vi "Main.vi"() -> ()   [LabVIEW 2011]
uses:
  Ch1.ctl
  <vilib>/DAQmx/write.llb/DAQmx Write (Analog DBL 1Chan 1Samp).vi
  <vilib>/DAQmx/read.llb/DAQmx Read (Analog DBL 1Chan 1Samp).vi
  <vilib>/DAQmx/write.llb/DAQmx Write (Digital Bool 1Line 1Point).vi
  <vilib>/DAQmx/read.llb/DAQmx Read (Digital Bool 1Line 1Point).vi
  <vilib>/DAQmx/create/channels.llb/DAQmx Create Channel (AO-Voltage-Basic).vi
  <vilib>/DAQmx/create/channels.llb/DAQmx Create Channel (AI-Voltage-Basic).vi
  <vilib>/DAQmx/create/channels.llb/DAQmx Create Channel (DO-Digital Output).vi
  <vilib>/DAQmx/create/channels.llb/DAQmx Create Channel (DI-Digital Input).vi
  <vilib>/DAQmx/miscellaneous.llb/DAQmx Fill In Error Info.vi
panel:
  out "P1.3":bool
  out "P1.2":bool
  out "P1.1":bool
  out "P1.0":bool
  in  "P0.3":bool
  in  "P0.2":bool
  in  "P0.1":bool
  in  "P0.0":bool
  out "U04, B":refnum<k21>
  out "U37, B":refnum<k21>
  out "U26, B":refnum<k21>
  out "U15, B":refnum<k21>
  in  "U1, B":dbl format="%0.2f"
  in  "U0, B":dbl format="%0.2f"
  in  "Зчитати з  P1.3":bool
  in  "Зчитати з  P1.2":bool
  in  "Зчитати з  P1.1":bool
  in  "Зчитати з  P1.0":bool
  in  "Записати в P0.3":bool
  in  "Записати в P0.2":bool
  in  "Записати в P0.1":bool
  in  "Записати в P0.0":bool
  in  "Зчитати з  Аl 37 (3)":bool
  in  "Зчитати з  Аl 26 (2)":bool
  in  "Зчитати з  Аl 15 (1)":bool
  in  "Зчитати з  Аl 04 (0)":bool
  in  "Записати в АО 1":bool
  in  "Записати в АО 0":bool
  in  "Exit":bool
  # "Аналогові канали"
  # "Цифрові канали"
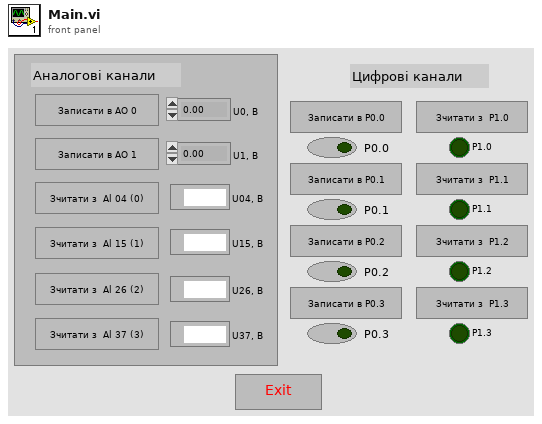
[diagram p1: front panel]
types:
  T1 = typedef "Ch1.ctl" = enum16{"def", "Exit", "Записати в АО 0", "Записати в АО 1", "Зчитати з  Аl 04 (0)", "Зчитати з  Аl 15 (1)", "Зчитати з  Аl 26 (2)", "Зчитати з  Аl 37 (3)", "Записати в P0.0", "Записати в  P0.1", "Записати в P0.2", "Записати в P0.3", "Зчитати з  P1.0", "Зчитати з  P1.1", "Зчитати з  P1.2", "Зчитати з  P1.3"}
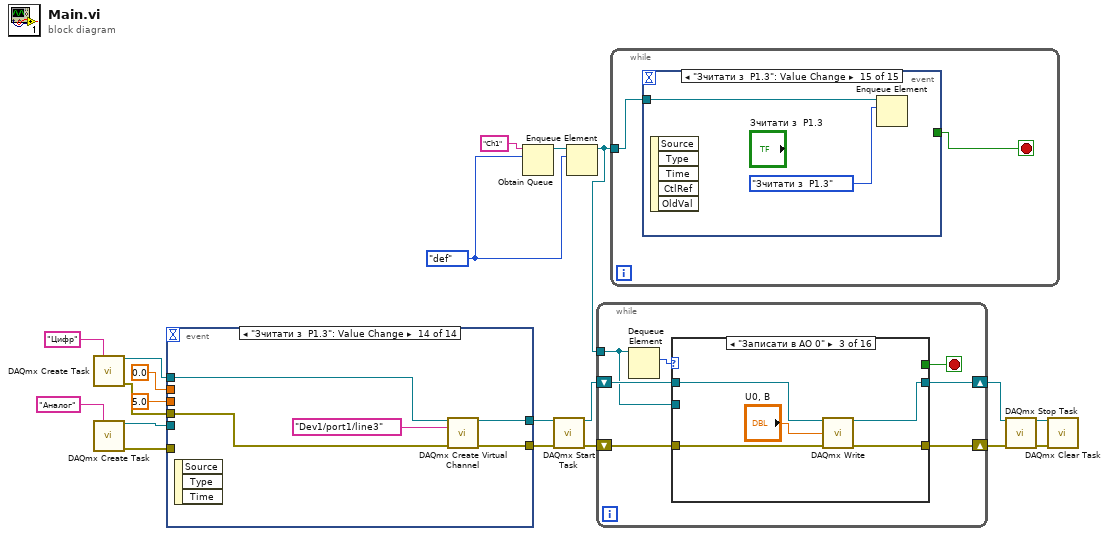
[diagram p0: block diagram]
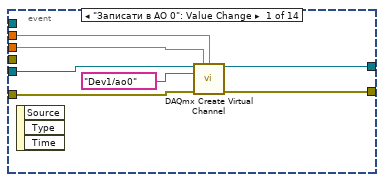
[diagram p2: hidden frame]
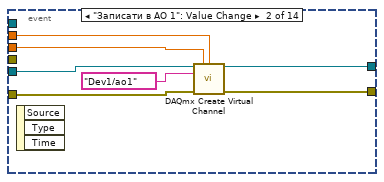
[diagram p3: hidden frame]
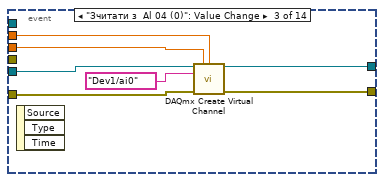
[diagram p4: hidden frame]
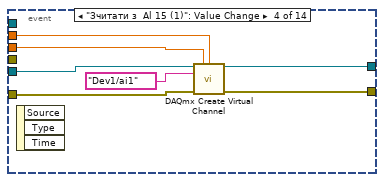
[diagram p5: hidden frame]
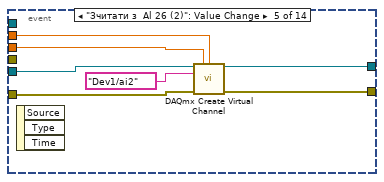
[diagram p6: hidden frame]
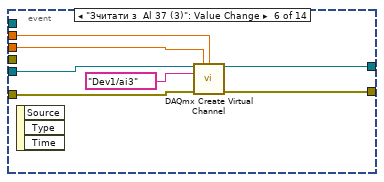
[diagram p7: hidden frame]
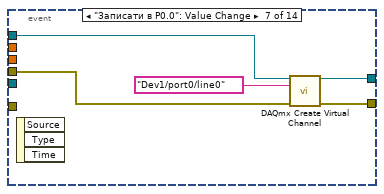
[diagram p8: hidden frame]
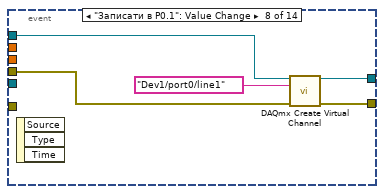
[diagram p9: hidden frame]
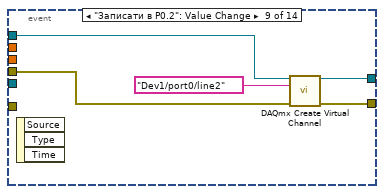
[diagram p10: hidden frame]
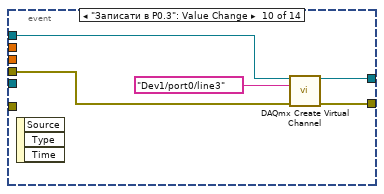
[diagram p11: hidden frame]
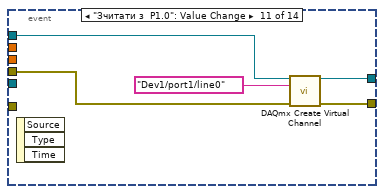
[diagram p12: hidden frame]
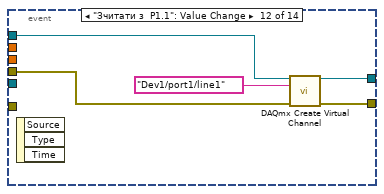
[diagram p13: hidden frame]
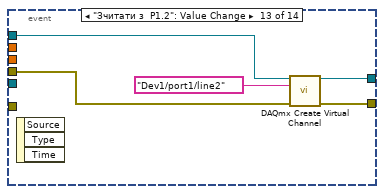
[diagram p14: hidden frame]
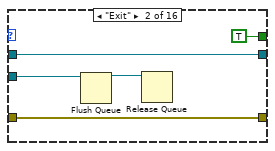
[diagram p16: hidden frame]
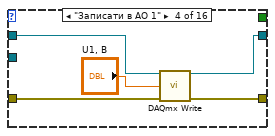
[diagram p17: hidden frame]
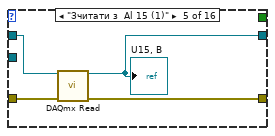
[diagram p18: hidden frame]
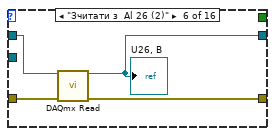
[diagram p19: hidden frame]
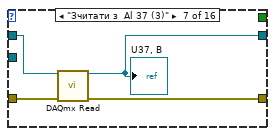
[diagram p20: hidden frame]
diagram:
  w20 = Ch1."def" ("Enum")
  n1 = call <vilib>:"DAQmx Create Task.vi"("new task name"="Цифр") -> ("task out"=w2:refnum<k21>, "error out"=w1:errorcluster)  [unwired: 13 in]
  n2 = call <vilib>:"DAQmx Create Task.vi"("new task name"="Аналог") -> ("task out"=w9:refnum<k21>, "error out"=w8:errorcluster)  [unwired: 13 in]
  n3 = event shown="[13] \"Зчитати з  P1.3\": Value Change" {
    selector: _ -> [_ _ _ _ _ _ _ _ _ _ _ _ _ _]
    dyn-events: _ -> [_ _ _ _ _ _ _ _ _ _ _ _ _ _]
    timeout: _ -> [_ _ _ _ _ _ _ _ _ _ _ _ _ _]
    tunnel: w9 -> [w26 w33 w41 w48 w55 w62 _ _ _ _ _ _ _ _]
    tunnel: w8 -> [w25 w32 w40 w47 w54 w61 _ _ _ _ _ _ _ _]
    tunnel: [w24 w31 w39 w46 w53 w60 w64 w69 w74 w79 w84 w89 w94 w99] -> w7
    tunnel: [w23 w30 w38 w45 w52 w59 w63 w68 w73 w78 w83 w88 w93 w98] -> w6
    tunnel: 0.0 ("minimum value") -> [w22 w29 w37 w44 w51 w58 _ _ _ _ _ _ _ _]
    tunnel: 5.0 ("maximum value") -> [w21 w28 w36 w43 w50 w57 _ _ _ _ _ _ _ _]
    tunnel: w2 -> [_ _ _ _ _ _ w66 w71 w76 w81 w86 w91 w96 w101]
    tunnel: w1 -> [_ _ _ _ _ _ w65 w70 w75 w80 w85 w90 w95 w100]
    event "Записати в АО 0": Value Change {
      n4 = event-data() -> ()  [unwired: 1 in, 3 out]
      n5 = call-poly <vilib>:"DAQmx Create Virtual Channel.vi"("task in"=w26, "maximum value"=w21, "minimum value"=w22, "physical channels"=tag "Dev1/ao0", "error in"=w25) -> ("task out"=w24:refnum<k21>, "error out"=w23:errorcluster)  [unwired: 9 in]
    }
    event "Записати в АО 1": Value Change {
      n6 = event-data() -> ()  [unwired: 1 in, 3 out]
      n7 = call-poly <vilib>:"DAQmx Create Virtual Channel.vi"("task in"=w33, "maximum value"=w28, "minimum value"=w29, "physical channels"=tag "Dev1/ao1", "error in"=w32) -> ("task out"=w31:refnum<k21>, "error out"=w30:errorcluster)  [unwired: 9 in]
    }
    event "Зчитати з  Аl 04 (0)": Value Change {
      n8 = event-data() -> ()  [unwired: 1 in, 3 out]
      n9 = call-poly <vilib>:"DAQmx Create Virtual Channel.vi"("task in"=w41, "maximum value"=w36, "minimum value"=w37, "physical channels"=tag "Dev1/ai0", "error in"=w40) -> ("task out"=w39:refnum<k21>, "error out"=w38:errorcluster)  [unwired: 9 in]
    }
    event "Зчитати з  Аl 15 (1)": Value Change {
      n10 = event-data() -> ()  [unwired: 1 in, 3 out]
      n11 = call-poly <vilib>:"DAQmx Create Virtual Channel.vi"("task in"=w48, "maximum value"=w43, "minimum value"=w44, "physical channels"=tag "Dev1/ai1", "error in"=w47) -> ("task out"=w46:refnum<k21>, "error out"=w45:errorcluster)  [unwired: 9 in]
    }
    event "Зчитати з  Аl 26 (2)": Value Change {
      n12 = event-data() -> ()  [unwired: 1 in, 3 out]
      n13 = call-poly <vilib>:"DAQmx Create Virtual Channel.vi"("task in"=w55, "maximum value"=w50, "minimum value"=w51, "physical channels"=tag "Dev1/ai2", "error in"=w54) -> ("task out"=w53:refnum<k21>, "error out"=w52:errorcluster)  [unwired: 9 in]
    }
    event "Зчитати з  Аl 37 (3)": Value Change {
      n14 = event-data() -> ()  [unwired: 1 in, 3 out]
      n15 = call-poly <vilib>:"DAQmx Create Virtual Channel.vi"("task in"=w62, "maximum value"=w57, "minimum value"=w58, "physical channels"=tag "Dev1/ai3", "error in"=w61) -> ("task out"=w60:refnum<k21>, "error out"=w59:errorcluster)  [unwired: 9 in]
    }
    event "Записати в P0.0": Value Change {
      n16 = event-data() -> ()  [unwired: 1 in, 3 out]
      n17 = call-poly <vilib>:"DAQmx Create Virtual Channel.vi"("task in"=w66, "lines"=tag "Dev1/port0/line0", "error in"=w65) -> ("task out"=w64:refnum<k21>, "error out"=w63:errorcluster)  [unwired: 11 in]
    }
    event "Записати в P0.1": Value Change {
      n18 = event-data() -> ()  [unwired: 1 in, 3 out]
      n19 = call-poly <vilib>:"DAQmx Create Virtual Channel.vi"("task in"=w71, "lines"=tag "Dev1/port0/line1", "error in"=w70) -> ("task out"=w69:refnum<k21>, "error out"=w68:errorcluster)  [unwired: 11 in]
    }
    event "Записати в P0.2": Value Change {
      n20 = event-data() -> ()  [unwired: 1 in, 3 out]
      n21 = call-poly <vilib>:"DAQmx Create Virtual Channel.vi"("task in"=w76, "lines"=tag "Dev1/port0/line2", "error in"=w75) -> ("task out"=w74:refnum<k21>, "error out"=w73:errorcluster)  [unwired: 11 in]
    }
    event "Записати в P0.3": Value Change {
      n22 = event-data() -> ()  [unwired: 1 in, 3 out]
      n23 = call-poly <vilib>:"DAQmx Create Virtual Channel.vi"("task in"=w81, "lines"=tag "Dev1/port0/line3", "error in"=w80) -> ("task out"=w79:refnum<k21>, "error out"=w78:errorcluster)  [unwired: 11 in]
    }
    event "Зчитати з  P1.0": Value Change {
      n24 = event-data() -> ()  [unwired: 1 in, 3 out]
      n25 = call-poly <vilib>:"DAQmx Create Virtual Channel.vi"("task in"=w86, "lines"=tag "Dev1/port1/line0", "error in"=w85) -> ("task out"=w84:refnum<k21>, "error out"=w83:errorcluster)  [unwired: 11 in]
    }
    event "Зчитати з  P1.1": Value Change {
      n26 = event-data() -> ()  [unwired: 1 in, 3 out]
      n27 = call-poly <vilib>:"DAQmx Create Virtual Channel.vi"("task in"=w91, "lines"=tag "Dev1/port1/line1", "error in"=w90) -> ("task out"=w89:refnum<k21>, "error out"=w88:errorcluster)  [unwired: 11 in]
    }
    event "Зчитати з  P1.2": Value Change {
      n28 = event-data() -> ()  [unwired: 1 in, 3 out]
      n29 = call-poly <vilib>:"DAQmx Create Virtual Channel.vi"("task in"=w96, "lines"=tag "Dev1/port1/line2", "error in"=w95) -> ("task out"=w94:refnum<k21>, "error out"=w93:errorcluster)  [unwired: 11 in]
    }
    event "Зчитати з  P1.3": Value Change {
      n30 = event-data() -> ()  [unwired: 1 in, 3 out]
      n31 = call-poly <vilib>:"DAQmx Create Virtual Channel.vi"("task in"=w101, "lines"=tag "Dev1/port1/line3", "error in"=w100) -> ("task out"=w99:refnum<k21>, "error out"=w98:errorcluster)  [unwired: 11 in]
    }
  }
  n32 = Obtain Queue(name (unnamed)="Ch1", element data type=w20) -> (queue out=w19:refnum<queue>)  [unwired: 3 in, 2 out]
  n33 = call <vilib>:"DAQmx Start Task.vi"("task/channels in"=w7, "error in"=w6) -> ("task out"=w15:refnum<k21>, "error out"=w14:errorcluster)  [unwired: 12 in]
  n34 = Enqueue Element(queue=w19, element=w20) -> (queue out=w17:refnum<queue>)  [unwired: 2 in, 2 out]
  n35 = while {
    tunnel: w17 -> [w103]
    shift-right: [w105] -> w11
    shift-left: w15 -> [w107]
    shift-right: [w104] -> w10
    shift-left: w14 -> [w106]
    stop <- w108 stop-if-true
    n36 = Dequeue Element(queue=w103) -> (element=w109:T1)  [unwired: 2 in, 3 out]
    n37 = case shown="\"Записати в АО 0\"" w109 {
      tunnel: [_ TRUE _ _ _ _ _ _ _ _ _ _ _ _ _ _] -> w108
      tunnel: w107 -> [w110 w115 w121 w126 w128 w133 w137 w143 w148 w153 w158 w161 w166 w171 w176 w181]
      tunnel: w106 -> [w111 w114 w120 w125 w129 w132 w136 w142 w147 w152 w157 w160 w165 w170 w175 w180]
      tunnel: [w110 w115 w119 w124 w127 w131 w135 w141 w146 w151 w156 w163 w168 w173 w178 w179] -> w105
      tunnel: [w111 w114 w118 w123 w130 w134 w138 w140 w145 w150 w155 w162 w167 w172 w177 w182] -> w104
      tunnel: w103 -> [_ w113 _ _ _ _ _ _ _ _ _ _ _ _ _ _]
      frame "def", Default {
      }
      frame "Exit" {
        n38 = Flush Queue(queue=w113) -> (queue out=w112:refnum<queue>)  [unwired: 1 in, 2 out]
        n39 = Release Queue(queue=w112) -> ()  [unwired: 2 in, 3 out]
      }
      frame "Записати в АО 0" {
        n40 = call-poly <vilib>:"DAQmx Write.vi"("task/channels in"=w121, "data"="U0, B", "error in"=w120) -> ("task out"=w119:refnum<k21>, "error out"=w118:errorcluster)  [unwired: 10 in, 1 out]
      }
      frame "Записати в АО 1" {
        n41 = call-poly <vilib>:"DAQmx Write.vi"("task/channels in"=w126, "data"="U1, B", "error in"=w125) -> ("task out"=w124:refnum<k21>, "error out"=w123:errorcluster)  [unwired: 10 in, 1 out]
      }
      frame "Зчитати з  Аl 15 (1)" {
        n42 = call-poly <vilib>:"DAQmx Read.vi"("task/channels in"=w128, "error in"=w129) -> ("task out"=w127:refnum<k21>, "error out"=w130:errorcluster)  [unwired: 11 in, 1 out]
        "U15, B" <- w127
      }
      frame "Зчитати з  Аl 26 (2)" {
        n43 = call-poly <vilib>:"DAQmx Read.vi"("task/channels in"=w133, "error in"=w132) -> ("task out"=w131:refnum<k21>, "error out"=w134:errorcluster)  [unwired: 11 in, 1 out]
        "U26, B" <- w131
      }
      frame "Зчитати з  Аl 37 (3)" {
        n44 = call-poly <vilib>:"DAQmx Read.vi"("task/channels in"=w137, "error in"=w136) -> ("task out"=w135:refnum<k21>, "error out"=w138:errorcluster)  [unwired: 11 in, 1 out]
        "U37, B" <- w135
      }
      frame "Записати в P0.0" {
        n45 = call-poly <vilib>:"DAQmx Write.vi"("task/channels in"=w143, "data"="P0.0", "error in"=w142) -> ("task out"=w141:refnum<k21>, "error out"=w140:errorcluster)  [unwired: 10 in, 1 out]
      }
      frame "Записати в  P0.1" {
        n46 = call-poly <vilib>:"DAQmx Write.vi"("task/channels in"=w148, "data"="P0.1", "error in"=w147) -> ("task out"=w146:refnum<k21>, "error out"=w145:errorcluster)  [unwired: 10 in, 1 out]
      }
      frame "Записати в P0.2" {
        n47 = call-poly <vilib>:"DAQmx Write.vi"("task/channels in"=w153, "data"="P0.2", "error in"=w152) -> ("task out"=w151:refnum<k21>, "error out"=w150:errorcluster)  [unwired: 10 in, 1 out]
      }
      frame "Записати в P0.3" {
        n48 = call-poly <vilib>:"DAQmx Write.vi"("task/channels in"=w158, "data"="P0.3", "error in"=w157) -> ("task out"=w156:refnum<k21>, "error out"=w155:errorcluster)  [unwired: 10 in, 1 out]
      }
      frame "Зчитати з  P1.0" {
        n49 = call-poly <vilib>:"DAQmx Read.vi"("task/channels in"=w161, "error in"=w160) -> ("task out"=w163:refnum<k21>, "data"=→"P1.0":bool, "error out"=w162:errorcluster)  [unwired: 11 in]
      }
      frame "Зчитати з  P1.1" {
        n50 = call-poly <vilib>:"DAQmx Read.vi"("task/channels in"=w166, "error in"=w165) -> ("task out"=w168:refnum<k21>, "data"=→"P1.1":bool, "error out"=w167:errorcluster)  [unwired: 11 in]
      }
      frame "Зчитати з  P1.2" {
        n51 = call-poly <vilib>:"DAQmx Read.vi"("task/channels in"=w171, "error in"=w170) -> ("task out"=w173:refnum<k21>, "data"=→"P1.2":bool, "error out"=w172:errorcluster)  [unwired: 11 in]
      }
      frame "Зчитати з  P1.3" {
        n52 = call-poly <vilib>:"DAQmx Read.vi"("task/channels in"=w176, "error in"=w175) -> ("task out"=w178:refnum<k21>, "data"=→"P1.3":bool, "error out"=w177:errorcluster)  [unwired: 11 in]
      }
      frame "Зчитати з  Аl 04 (0)" {
        n53 = call-poly <vilib>:"DAQmx Read.vi"("task/channels in"=w181, "error in"=w180) -> ("task out"=w179:refnum<k21>, "error out"=w182:errorcluster)  [unwired: 11 in, 1 out]
        "U04, B" <- w179
      }
    }
  }
  n54 = while {
    tunnel: w17 -> [w184]
    stop <- w183 stop-if-true
    n55 = event shown="[14] \"Зчитати з  P1.3\": Value Change" {
      selector: _ -> [_ _ _ _ _ _ _ _ _ _ _ _ _ _ _]
      dyn-events: _ -> [_ _ _ _ _ _ _ _ _ _ _ _ _ _ _]
      timeout: _ -> [_ _ _ _ _ _ _ _ _ _ _ _ _ _ _]
      tunnel: w184 -> [w187 w189 w191 w193 w195 w197 w198 w200 w202 w204 w206 w208 w210 w212 w214]
      tunnel: [TRUE _ _ _ _ _ _ _ _ _ _ _ _ _ _] -> w183
      event "Exit": Value Change {
        n56 = event-data() -> ()  [unwired: 1 in, 5 out]
        n57 = Enqueue Element At Opposite End(queue=w187, element=Ch1."Exit" ("Enum")) -> ()  [unwired: 2 in, 3 out]
      }
      event "Записати в АО 0": Value Change {
        n58 = event-data() -> ()  [unwired: 1 in, 5 out]
        n59 = Enqueue Element(queue=w189, element=Ch1."Записати в АО 0" ("Enum")) -> ()  [unwired: 2 in, 3 out]
      }
      event "Зчитати з  Аl 04 (0)": Value Change {
        n60 = event-data() -> ()  [unwired: 1 in, 5 out]
        n61 = Enqueue Element(queue=w191, element=Ch1."Зчитати з  Аl 04 (0)" ("Enum")) -> ()  [unwired: 2 in, 3 out]
      }
      event "Зчитати з  Аl 15 (1)": Value Change {
        n62 = event-data() -> ()  [unwired: 1 in, 5 out]
        n63 = Enqueue Element(queue=w193, element=Ch1."Зчитати з  Аl 15 (1)" ("Enum")) -> ()  [unwired: 2 in, 3 out]
      }
      event "Зчитати з  Аl 26 (2)": Value Change {
        n64 = event-data() -> ()  [unwired: 1 in, 5 out]
        n65 = Enqueue Element(queue=w195, element=Ch1."Зчитати з  Аl 26 (2)" ("Enum")) -> ()  [unwired: 2 in, 3 out]
      }
      event "Зчитати з  Аl 37 (3)": Value Change {
        n66 = event-data() -> ()  [unwired: 1 in, 5 out]
        n67 = Enqueue Element(queue=w197, element=Ch1."Зчитати з  Аl 37 (3)" ("Enum")) -> ()  [unwired: 2 in, 3 out]
      }
      event "Записати в АО 1": Value Change {
        n68 = event-data() -> ()  [unwired: 1 in, 5 out]
        n69 = Enqueue Element(queue=w198, element=Ch1."Записати в АО 1" ("Enum")) -> ()  [unwired: 2 in, 3 out]
      }
      event "Записати в P0.0": Value Change {
        n70 = event-data() -> ()  [unwired: 1 in, 5 out]
        n71 = Enqueue Element(queue=w200, element=Ch1."Записати в P0.0" ("Enum")) -> ()  [unwired: 2 in, 3 out]
      }
      event "Записати в P0.1": Value Change {
        n72 = event-data() -> ()  [unwired: 1 in, 5 out]
        n73 = Enqueue Element(queue=w202, element=Ch1."Записати в  P0.1" ("Enum")) -> ()  [unwired: 2 in, 3 out]
      }
      event "Записати в P0.2": Value Change {
        n74 = event-data() -> ()  [unwired: 1 in, 5 out]
        n75 = Enqueue Element(queue=w204, element=Ch1."Записати в P0.2" ("Enum")) -> ()  [unwired: 2 in, 3 out]
      }
      event "Записати в P0.3": Value Change {
        n76 = event-data() -> ()  [unwired: 1 in, 5 out]
        n77 = Enqueue Element(queue=w206, element=Ch1."Записати в P0.3" ("Enum")) -> ()  [unwired: 2 in, 3 out]
      }
      event "Зчитати з  P1.0": Value Change {
        n78 = event-data() -> ()  [unwired: 1 in, 5 out]
        n79 = Enqueue Element(queue=w208, element=Ch1."Зчитати з  P1.0" ("Enum")) -> ()  [unwired: 2 in, 3 out]
      }
      event "Зчитати з  P1.1": Value Change {
        n80 = event-data() -> ()  [unwired: 1 in, 5 out]
        n81 = Enqueue Element(queue=w210, element=Ch1."Зчитати з  P1.1" ("Enum")) -> ()  [unwired: 2 in, 3 out]
      }
      event "Зчитати з  P1.2": Value Change {
        n82 = event-data() -> ()  [unwired: 1 in, 5 out]
        n83 = Enqueue Element(queue=w212, element=Ch1."Зчитати з  P1.2" ("Enum")) -> ()  [unwired: 2 in, 3 out]
      }
      event "Зчитати з  P1.3": Value Change {
        n84 = event-data() -> ()  [unwired: 1 in, 5 out]
        n85 = Enqueue Element(queue=w214, element=Ch1."Зчитати з  P1.3" ("Enum")) -> ()  [unwired: 2 in, 3 out]
      }
    }
  }
  n86 = call <vilib>:"DAQmx Stop Task.vi"("task/channels in"=w11, "error in"=w10) -> ("task out"=w12:refnum<k21>, "error out"=w13:errorcluster)  [unwired: 12 in]
  n87 = call <vilib>:"DAQmx Clear Task.vi"("task in"=w12, "error in"=w13) -> ()  [unwired: 13 in, 1 out]
